vi "ToString.vi"(0 "reference in":refnum<class "Cylinder.lvclass">, 5 "error in (no error)":errorcluster) -> (14 "reference out":refnum<class "Cylinder.lvclass">, 15 "string":string, 19 "error out":errorcluster)   [LabVIEW 2013, in "Cylinder.lvclass"]
doc: "Defines a method that allows a class to return one string as a representation of the object."
uses:
  Cylinder.lvclass
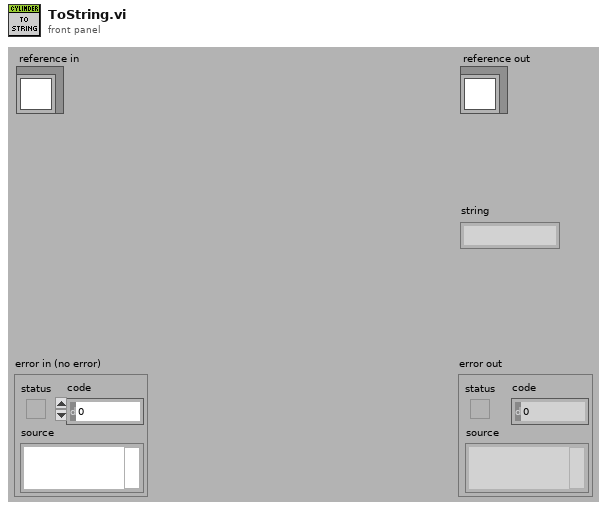
[diagram p1: front panel]
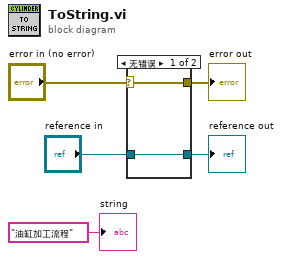
[diagram p0: block diagram]
diagram:
  n1 = case shown="无错误" "error in (no error)" {
    selector: "error in (no error)" -> [w6 w9]
    tunnel: [w6 w9] -> w4
    tunnel: [w7 w8] -> w2
    tunnel: "reference in" -> [w7 w8]
    frame No Error {
    }
    frame Error {
    }
  }
  "error out" <- w4
  "reference out" <- w2
  "string" <- "油缸加工流程" ("string")
